vi "Next Step.vi"(8 "error in (no error)":errorcluster, 11 "AutomationContext in":refnum<class "AutomationContext.lvclass">) -> (0 "error out":errorcluster, 3 "AutomationContext out":refnum<class "AutomationContext.lvclass">)   [LabVIEW 2023, in "Automation.lvlib" / "AutomationContext.lvclass"]
uses:
  AutomationContext.lvclass
  AutomationContext.lvclass/AutomationContext.ctl
  Application Messages/Stage Forward Msg/Stage Forward Msg.lvclass/Stage Forward Msg.ctl
  <vilib>/ActorFramework/Message Enqueuer/Message Enqueuer.lvclass/Message Enqueuer.ctl
  Application Messages/Stage Previous Lane Msg/Stage Previous Lane Msg.lvclass/Stage Previous Lane Msg.ctl
  Application Messages/Set All Laser Powers Msg/Set All Laser Powers Msg.lvclass/Set All Laser Powers Msg.ctl
  Application Messages/Reset Laser Power Msg/Reset Laser Power Msg.lvclass/Reset Laser Power Msg.ctl
  Application Messages/Start Autofocus Msg/Start Autofocus Msg.lvclass/Start Autofocus Msg.ctl
  Resources/Type Defs/Camera Settings.ctl
  Application Messages/Start Stream Msg/Start Stream Msg.lvclass/Start Stream Msg.ctl
  <vilib>/ActorFramework/Message Enqueuer/Enqueue.vi
  Application Messages/Stage Forward Msg/Stage Forward Msg.lvclass
  Application Messages/Stage Previous Lane Msg/Stage Previous Lane Msg.lvclass
  Application Messages/Set All Laser Powers Msg/Set All Laser Powers Msg.lvclass
  Application Messages/Reset Laser Power Msg/Reset Laser Power Msg.lvclass
  Application Messages/Start Autofocus Msg/Start Autofocus Msg.lvclass
  Application Messages/Start Stream Msg/Start Stream Msg.lvclass
  Application Messages/Finish Recording Msg/Finish Recording Msg.lvclass
  <vilib>/ActorFramework/Message Priority Queue/Priority Enqueue.vi
  Application Messages/Open Shutter Msg/Open Shutter Msg.lvclass
  Application Messages/Close Shutter Msg/Close Shutter Msg.lvclass
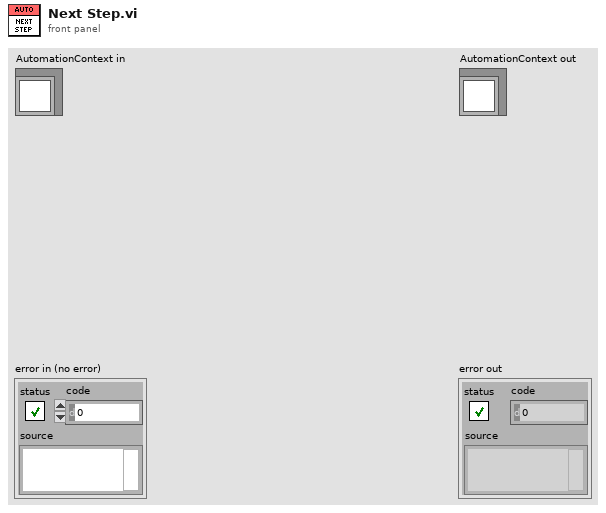
[diagram p1: front panel]
types:
  T1 = typedef "Camera Settings.ctl" = cluster{"Exposure Time (ms)":dbl, "Binning":enum16{"1x1", "2x2", "4x4"}, "Scan Mode":i32, "Frames to Acquire":dbl, "Pixel Correction":bool, "Frames to Skip":u32, "File Path":path, "Duty cycle":dbl, "ALEX":bool, "Shutter Enable":bool[], "fluidics trigger, ms (0=disabled)":dbl, "Bit Depth":u16, "Image Width (px)":u16, "Image Height (px)":u16, "Horizontal Offset (px)":u16, "Vertical Offset (px)":u16}
  T2 = cluster{"Camera Settings":T1, "Injection Countdown":bool}
  T3 = typedef "Automation.lvlib/AutomationContext.lvclass/Automation Intent.ctl" = cluster{"Action":T4, "Parameters":variant, "Correlation ID":u32}
  T4 = typedef "Automation.lvlib/AutomationContext.lvclass/Intent Action.ctl" = enum16{"Next Field", "Next Lane", "Set Power", "Reset Power", "Autofocus", "Start Streaming", "Delay", "Finish Run", "Open Shutter", "Close Shutter"}
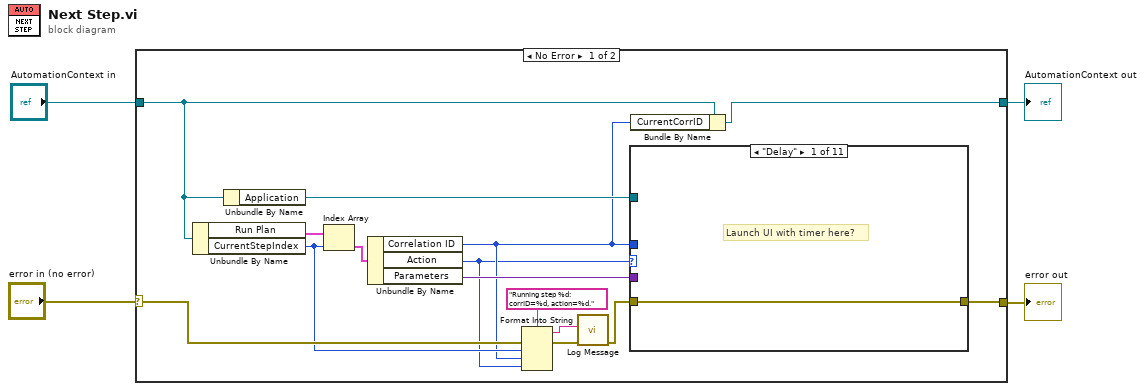
[diagram p0: block diagram]
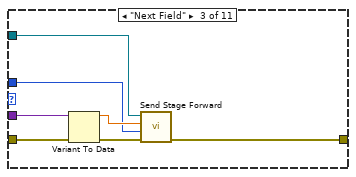
[diagram p3: hidden frame]
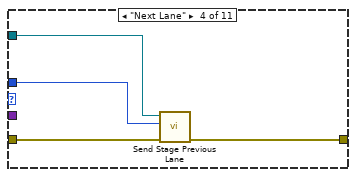
[diagram p4: hidden frame]
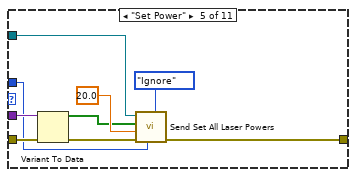
[diagram p5: hidden frame]
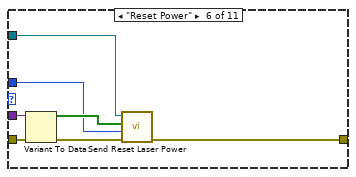
[diagram p6: hidden frame]
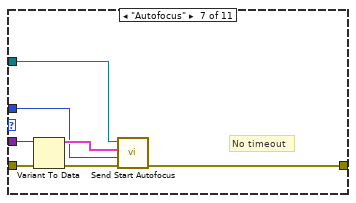
[diagram p7: hidden frame]
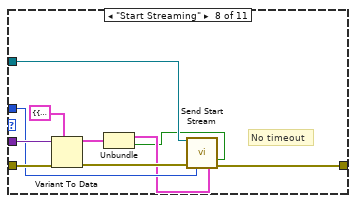
[diagram p8: hidden frame]
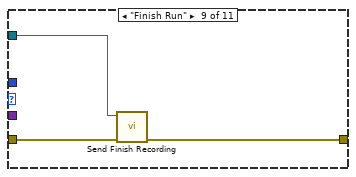
[diagram p9: hidden frame]
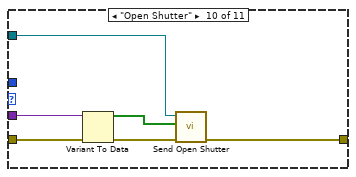
[diagram p10: hidden frame]
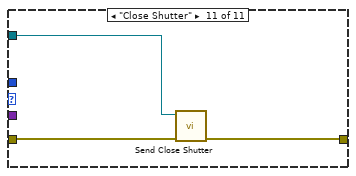
[diagram p11: hidden frame]
diagram:
  n1 = case shown="No Error" "error in (no error)" {
    selector: "error in (no error)" -> [w9 w79]
    tunnel: [w14 w79] -> w3
    tunnel: [w12 w78] -> w1
    tunnel: "AutomationContext in" -> [w13 w78]
    frame No Error {
      n2 = Unbundle By Name(w13) -> ("Run Plan"=w19:T3[], "CurrentStepIndex"=w8:u32)
      n3 = Unbundle By Name(w13) -> ("Application"=w17:refnum<class "Message Enqueuer.lvclass">)
      n4 = Index Array(array=w19, index=w8) -> (element=w15:T3)
      n5 = Unbundle By Name(w15) -> ("Correlation ID"=w6:u32, "Action"=w5:T4, "Parameters"=w18:variant)
      n6 = Format Into String(format string="Running step %d: corrID=%d, action=%d." ("input"), error in=w9, w8, w6, w5) -> (resulting string=w11:string, error out=w10:errorcluster)  [unwired: 1 in]
      n7 = call "Log Message.vi"("error constant"=w10, "input"=w11) -> ("error constant 2"=w16:errorcluster)  [unwired: 8 in, 1 out]
      n8 = case shown="\"Delay\"" w5 {
        tunnel: w16 -> [w20 w21 w26 w32 w40 w47 w53 w64 w68 w72 w77]
        tunnel: w18 -> [_ _ w27 _ w39 w45 w51 w62 _ w70 _]
        tunnel: [w20 w21 w23 w29 w35 w42 w55 w59 w67 w74 w76] -> w14
        tunnel: w17 -> [_ _ w28 w31 w41 w48 w54 w65 w66 w73 w75]
        tunnel: w6 -> [_ _ w22 w30 w33 w43 w49 w58 _ _ _]
        frame "Delay" {
          # "Launch UI with timer here?"
        }
        frame Default {
        }
        frame "Next Field" {
          n9 = Variant To Data(error in=w26, Variant=w27) -> (data=w24:dbl, error out=w25:errorcluster)  [unwired: 1 in]
          n10 = call "Send Stage Forward.vi"("error in (no error)"=w25, "Correlation ID"=w22, "Multiple"=w24, "Message Enqueuer"=w28) -> ("error out"=w23:errorcluster)  [unwired: 6 in, 1 out]
        }
        frame "Next Lane" {
          n11 = call "Send Stage Previous Lane.vi"("error in (no error)"=w32, "Correlation ID"=w30, "Message Enqueuer"=w31) -> ("error out"=w29:errorcluster)  [unwired: 7 in, 1 out]
        }
        frame "Set Power" {
          n12 = Variant To Data(error in=w40, Variant=w39) -> (data=w36:bool[], error out=w38:errorcluster)  [unwired: 1 in]
          n13 = call "Send Set All Laser Powers.vi"("Mode"=enum16{"Normal", "Ignore", "Reset"}."Ignore", "Correlation ID"=w33, "error in (no error)"=w38, "Power"=20.0, "Line Enable"=w36, "Message Enqueuer"=w41) -> ("error out"=w35:errorcluster)  [unwired: 4 in, 1 out]
        }
        frame "Reset Power" {
          n14 = Variant To Data(error in=w47, Variant=w45) -> (data=w44:bool[], error out=w46:errorcluster)  [unwired: 1 in]
          n15 = call "Send Reset Laser Power.vi"("error in (no error)"=w46, "Correlation ID"=w43, "Shutter Enable"=w44, "Message Enqueuer"=w48) -> ("error out"=w42:errorcluster)  [unwired: 6 in, 1 out]
        }
        frame "Autofocus" {
          # "No timeout"
          n16 = Variant To Data(error in=w53, Variant=w51) -> (data=w50:T1, error out=w52:errorcluster)  [unwired: 1 in]
          n17 = call "Send Start Autofocus.vi"("error in (no error)"=w52, "Correlation ID"=w49, "Camera Settings"=w50, "Message Enqueuer"=w54) -> ("error out"=w55:errorcluster)  [unwired: 6 in, 1 out]
        }
        frame "Start Streaming" {
          # "No timeout"
          n18 = Variant To Data(error in=w64, type=T2 {"Camera Settings"={"Exposure Time (ms)"=0.0, "Binning"=enum."1x1", "Scan Mode"=0, "Frames to Acquire"=0.0, "Pixel Correction"=FALSE, "Frames to Skip"=0, "File Path"=path "", "Duty cycle"=0.0, "ALEX"=FALSE, "Shutter Enable"=[], "fluidics trigger, ms (0=disabled)"=0.0, "Bit Depth"=0, "Image Width (px)"=0, "Image Height (px)"=0, "Horizontal Offset (px)"=0, "Vertical Offset (px)"=0}, "Injection Countdown"=FALSE} ("cluster"), Variant=w62) -> (data=w60:T2, error out=w63:errorcluster)
          n19 = Unbundle(w60) -> ("Camera Settings"=w57:T1, "Injection Countdown"=w56:bool)
          n20 = call "Send Start Stream.vi"("Message Enqueuer"=w65, "Injection Countdown"=w56, "error in (no error)"=w63, "Correlation ID"=w58, "Camera Settings"=w57) -> ("error out"=w59:errorcluster)  [unwired: 9 in, 1 out]
        }
        frame "Finish Run" {
          n21 = call "Send Finish Recording.vi"("error in (no error)"=w68, "Message Enqueuer"=w66) -> ("error out"=w67:errorcluster)  [unwired: 8 in, 1 out]
        }
        frame "Open Shutter" {
          n22 = Variant To Data(error in=w72, Variant=w70) -> (data=w69:bool[], error out=w71:errorcluster)  [unwired: 1 in]
          n23 = call "Send Open Shutter.vi"("error in (no error)"=w71, "Array"=w69, "Message Enqueuer"=w73) -> ("error out"=w74:errorcluster)  [unwired: 7 in, 1 out]
        }
        frame "Close Shutter" {
          n24 = call "Send Close Shutter.vi"("error in (no error)"=w77, "Message Enqueuer"=w75) -> ("error out"=w76:errorcluster)  [unwired: 8 in, 1 out]
        }
      }
      n25 = Bundle By Name(cluster=w13, "CurrentCorrID"=w6) -> (w12:refnum<class "AutomationContext.lvclass">)
    }
    frame Error {
    }
  }
  "error out" <- w3
  "AutomationContext out" <- w1
